vi "Create Guest History Map.vi"(11 "error in (no error)":errorcluster) -> (4 "Guest History Map":map{string, T1}(c390), 15 "error out":errorcluster)   [LabVIEW 2023, in "File Data Manager.lvlib" / "File Data Manager.lvclass"]
uses:
  File Data Manager.lvclass
  Central Data Manager/Central Data Manager/Guest Details.ctl
  File Data Manager.lvclass/File Data Manager.ctl
  <vilib>/Utility/file.llb/Read Delimited Spreadsheet (string).vi
  Utilities/Utilities.lvlib
  Central Data Manager/Central Data Manager/Central Data Manager.lvclass
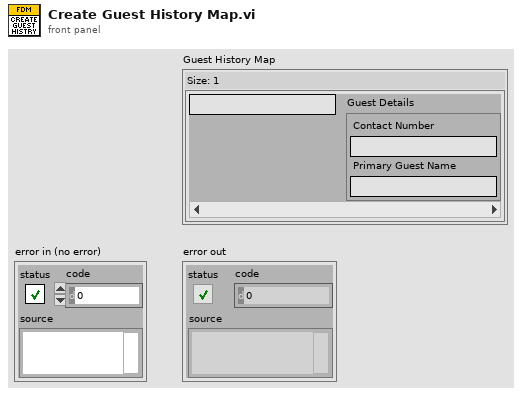
[diagram p1: front panel]
types:
  T1 = typedef "Central Data Manager.lvlib/Central Data Manager.lvclass/Guest Details.ctl" = cluster{"Contact Number":string, "Primary Guest Name":string}
  T2 = typedef "Hotel Management Tool Model.lvlib/Hotel Management Tool Model.lvclass/Database File Paths.ctl" = cluster{"Food Menu File Path":path, "Guests Histroy File Path":path, "Room Size File Path":path, "Rooms List File Path":path, "Rooms Service Allocation File Path":path, "Staff List File Path":path}
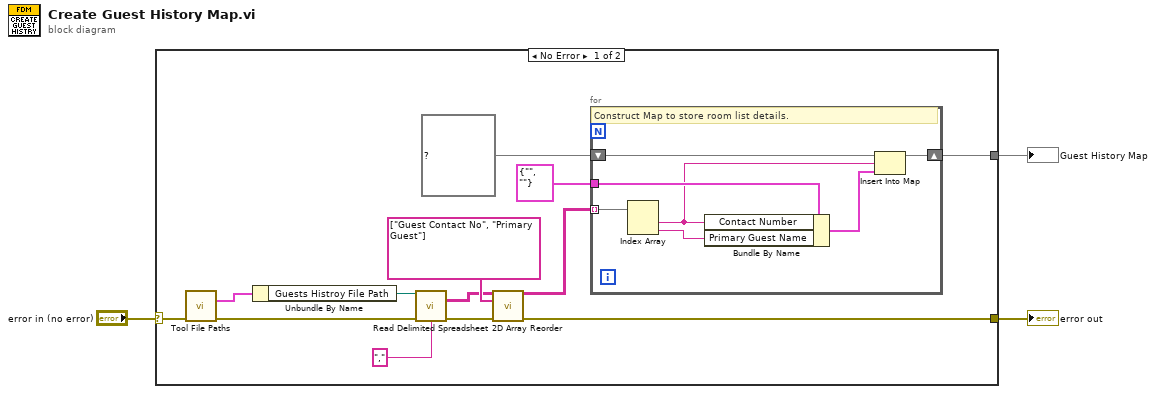
[diagram p0: block diagram]
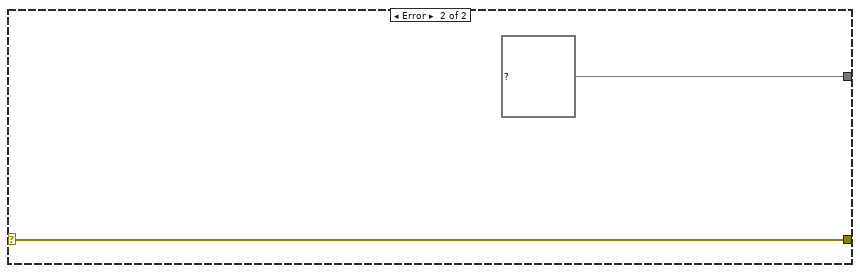
[diagram p2: hidden frame]
diagram:
  n1 = case shown="No Error" "error in (no error)" {
    selector: "error in (no error)" -> [w9 w25]
    tunnel: [w6 w25] -> w2
    tunnel: [w5 map{string, T1} {} ("Rooms List")] -> w1
    frame No Error {
      n2 = call "Tool File Paths.vi"("error in (no error)"=w9) -> ("Database File Paths"=w16:T2, "error out"=w15:errorcluster)  [unwired: 12 in, 1 out]
      n3 = Unbundle By Name(w16) -> ("Guests Histroy File Path"=w14:path)
      n4 = call-poly <vilib>:"Read Delimited Spreadsheet.vi"("file path (dialog if empty)"=w14, "error in (no error)"=w15, "delimiter (\\t)"="," ("delimiter (\\t)")) -> ("all rows"=w10:string[][], "error out"=w11:errorcluster)  [unwired: 7 in, 4 out]
      n5 = call "2D Array Reorder.vi"("2D Array Data witjh Header"=w10, "Header Order"=string[] ["Guest Contact No", "Primary Guest"] ("first row"), "error in (no error)"=w11) -> ("Reordered Data without Header"=w7:string[][], "error out"=w6:errorcluster)  [unwired: 11 in]
      n6 = for {
        tunnel: w7 -> [w20] mode=indexing
        shift-right: [w22] -> w5
        shift-left: map{string, T1} {} ("Rooms List") -> [w23]
        tunnel: T1 {"Contact Number"="", "Primary Guest Name"=""} ("Guest Details") -> [w21]
        # "Construct Map to store room list details."
        n7 = Index Array(array=w20) -> (element #1=w19:string, element #2=w17:string)  [unwired: 2 in]
        n8 = Bundle By Name(cluster=w21, "Contact Number"=w19, "Primary Guest Name"=w17) -> (w18:T1)
        n9 = Insert Into Map(map in=w23, key=w19, value=w18) -> (map out=w22:map{string, T1})  [unwired: 2 out]
      }
    }
    frame Error {
    }
  }
  "error out" <- w2
  "Guest History Map" <- w1
